vi "Begin.vi"(8 "error in":errorcluster) -> (0 "error out":errorcluster)   [LabVIEW 2018]
doc: "Called before other user functions, this VI can be used to open I/O refnums, load in file data, and do general program initialization. Notice that the <B>error out</B> terminal is simply used for data flow. Wiring it to other structures or subVIs ensures that this VI runs first."
uses:
  <vilib>/Rock Robotics/WPI/DriverStation/WPI_DriverStationRobotMode2.ctl
  <vilib>/Rock Robotics/WPI/Joystick/WPI_JoystickDeviceEnum.ctl
  <vilib>/Rock Robotics/WPI/ThirdParty/Phoenix-LabVIEW/Motor Controller/Controls/CTRE_Phoenix_MotorControl_ControlMode.ctl
  <vilib>/Rock Robotics/WPI/ThirdParty/Phoenix-LabVIEW/Motor Controller/Controls/CTRE_Phoenix_MotorControl_FeedbackDevice.ctl
  <vilib>/Rock Robotics/WPI/ThirdParty/Phoenix-LabVIEW/Motor Controller/Controls/CTRE_Phoenix_MotorControl_NeutralMode.ctl
  <vilib>/Rock Robotics/WPI/SafetyOutput/WPI_SafetyOutputConfigMenu.ctl
  <vilib>/Rock Robotics/SystemInterfaces/DIO/FPGA_DIOChannel.ctl
  Robot Global Data.vi
  <vilib>/Rock Robotics/Network Tables/NT Write String Array.vi
  <vilib>/Rock Robotics/WPI/RobotDrive/WPI_RobotDriveOpen4MotorWithExistingMotors.vi
  <vilib>/Rock Robotics/WPI/RobotDrive/WPI_RobotDriveOpen2MotorWithExistingMotors.vi
  <vilib>/Rock Robotics/WPI/Solenoid/WPI_SolenoidOpenDouble.vi
  <vilib>/Rock Robotics/WPI/Utilities/WPI_GetSetVariantRefNum.vi
  <vilib>/Rock Robotics/WPI/Solenoid/WPI_SolenoidOpenSingle.vi
  <vilib>/Rock Robotics/WPI/Ultrasonic/WPI_SonarSRF04DigitalOpen.vi
  <vilib>/Rock Robotics/WPI/Ultrasonic/WPI_SonarSRF04DigitalRefNum Registry Set.vi
  <vilib>/Rock Robotics/WPI/Switch/WPI_SwitchOpenLimit.vi
panel:
  in  "error in 2":errorcluster
  out "error out 2":errorcluster
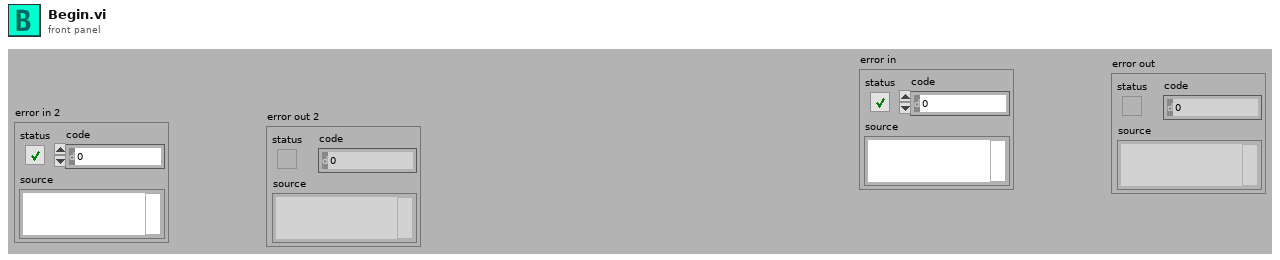
[diagram p1: front panel]
types:
  T1 = typedef "FPGA_DIOChannel.ctl" = enum8{"DIO 0", "DIO 1", "DIO 2", "DIO 3", "DIO 4", "DIO 5", "DIO 6", "DIO 7", "DIO 8", "DIO 9", "DIO MXP 0", "DIO MXP 1", "DIO MXP 2", "DIO MXP 3", "DIO MXP 4", "DIO MXP 5", "DIO MXP 6", "DIO MXP 7", "DIO MXP 8", "DIO MXP 9", "DIO MXP 10", "DIO MXP 11", "DIO MXP 12", "DIO MXP 13", "DIO MXP 14", "DIO MXP 15", "SPI Port CS1", "SPI Port CS2", "SPI Port CS3", "SPI Port MISO", "SPI Port MOSI", "Invalid"}
  T2 = typedef "CTRE_Phoenix_MotorControl_ControlMode.ctl" = u16
  T3 = typedef "WPI_SafetyOutputConfigMenu.ctl" = enum16{"Enable", "Disable"}
  T4 = typedef "WPI_JoystickDeviceEnum.ctl" = enum16{"USB 0", "USB 1", "USB 2", "USB 3", "USB 4", "USB 5"}
  T5 = typedef "CTRE_Phoenix_MotorControl_FeedbackDevice.ctl" = i8
  T6 = typedef "CTRE_Phoenix_MotorControl_NeutralMode.ctl" = enum8{"EEPROMSetting", "Override to Coast", "Override to Brake"}
  T7 = typedef "WPI_DriverStationRobotMode2.ctl" = enum16{"Autonomous Disabled", "Autonomous Enabled", "Teleop Disabled", "Teleop Enabled", "Disconnected", "Finish", "Test Disabled", "Test Enabled", "Emergency Stopped"}
  T8 = typedef "WPI_MotorControlDeviceRef.ctl" = cluster{"DeviceStatus":errorcluster, "Type":T9, "PWM":cluster{"PWM Channel":T10, "DeadBand":T11}, "CAN":cluster{"Device Number":u8, "SetOutput VI Ref":variant, "GetOutput VI Ref":variant, "Enable VI Ref":variant, "Disable VI Ref":variant, "Data":variant}, "Invert":bool, "DIO PWM":cluster{"PWM \"Enable\" Channel":T10, "DIOChannel":T1, "PWM Rate":dbl}}
  T9 = typedef "WPI_MotorControlType.ctl" = enum16{"PWM", "CAN", "DIO PWM"}
  T10 = typedef "FPGA_DIOPWMChannel.ctl" = enum8{"PWM 0", "PWM 1", "PWM 2", "PWM 3", "PWM 4", "PWM 5", "PWM 6", "PWM 7", "PWM 8", "PWM 9", "PWM MXP 0", "PWM MXP 1", "PWM MXP 2", "PWM MXP 3", "PWM MXP 4", "PWM MXP 5", "PWM MXP 6", "PWM MXP 7", "PWM MXP 8", "PWM MXP 9", "Invalid"}
  T11 = typedef "WPI_PWMDeadband.ctl" = cluster{"Name":string, "maxPositivePwm":i32, "minPositivePwm":i32, "centerPwm":i32, "maxNegativePwm":i32, "minNegativePwm":i32, "angularRange":u16}
  T12 = typedef "WPI_JoystickDevRef.ctl" = cluster{"Device":T4}
  T13 = typedef "WPI_CompressorDevRef.ctl" = cluster{"DevStatus":errorcluster, "Pneumatics Control Module":u8}
  T14 = typedef "WPI_SwitchDevRef.ctl" = cluster{"DevStatus":errorcluster, "DIO Channel":T1, "CntIndex":T15, "Normally Closed":bool}
  T15 = typedef "FPGA_CounterCtrSystemIndex.ctl" = enum8{"Ctr 0", "Ctr 1", "Ctr 2", "Ctr 3", "Ctr 4", "Ctr 5", "Ctr 6", "Ctr 7", "Invalid"}
  T16 = typedef "WPI_SolenoidDevRef.ctl" = cluster{"DevStatus":errorcluster, "Pneumatics Control Module":u8, "Forward Solenoid Channel":T17, "Reverse Solenoid Channel":T17}
  T17 = typedef "WPI_SolenoidChannel.ctl" = enum8{"Solenoid 0", "Solenoid 1", "Solenoid 2", "Solenoid 3", "Solenoid 4", "Solenoid 5", "Solenoid 6", "Solenoid 7", "Invalid"}
  T18 = typedef "WPI_RobotDriveDevRef.ctl" = cluster{"DevStatus":errorcluster, "Motors[]":T8[], "Square Inputs":bool, "Max Output":dbl}
  T19 = typedef "WPI_UltrasonicDeviceRef.ctl" = cluster{"DevStatus":errorcluster, "Ping Channel":T1, "Echo Channel":T1, "CntIndex":T15}
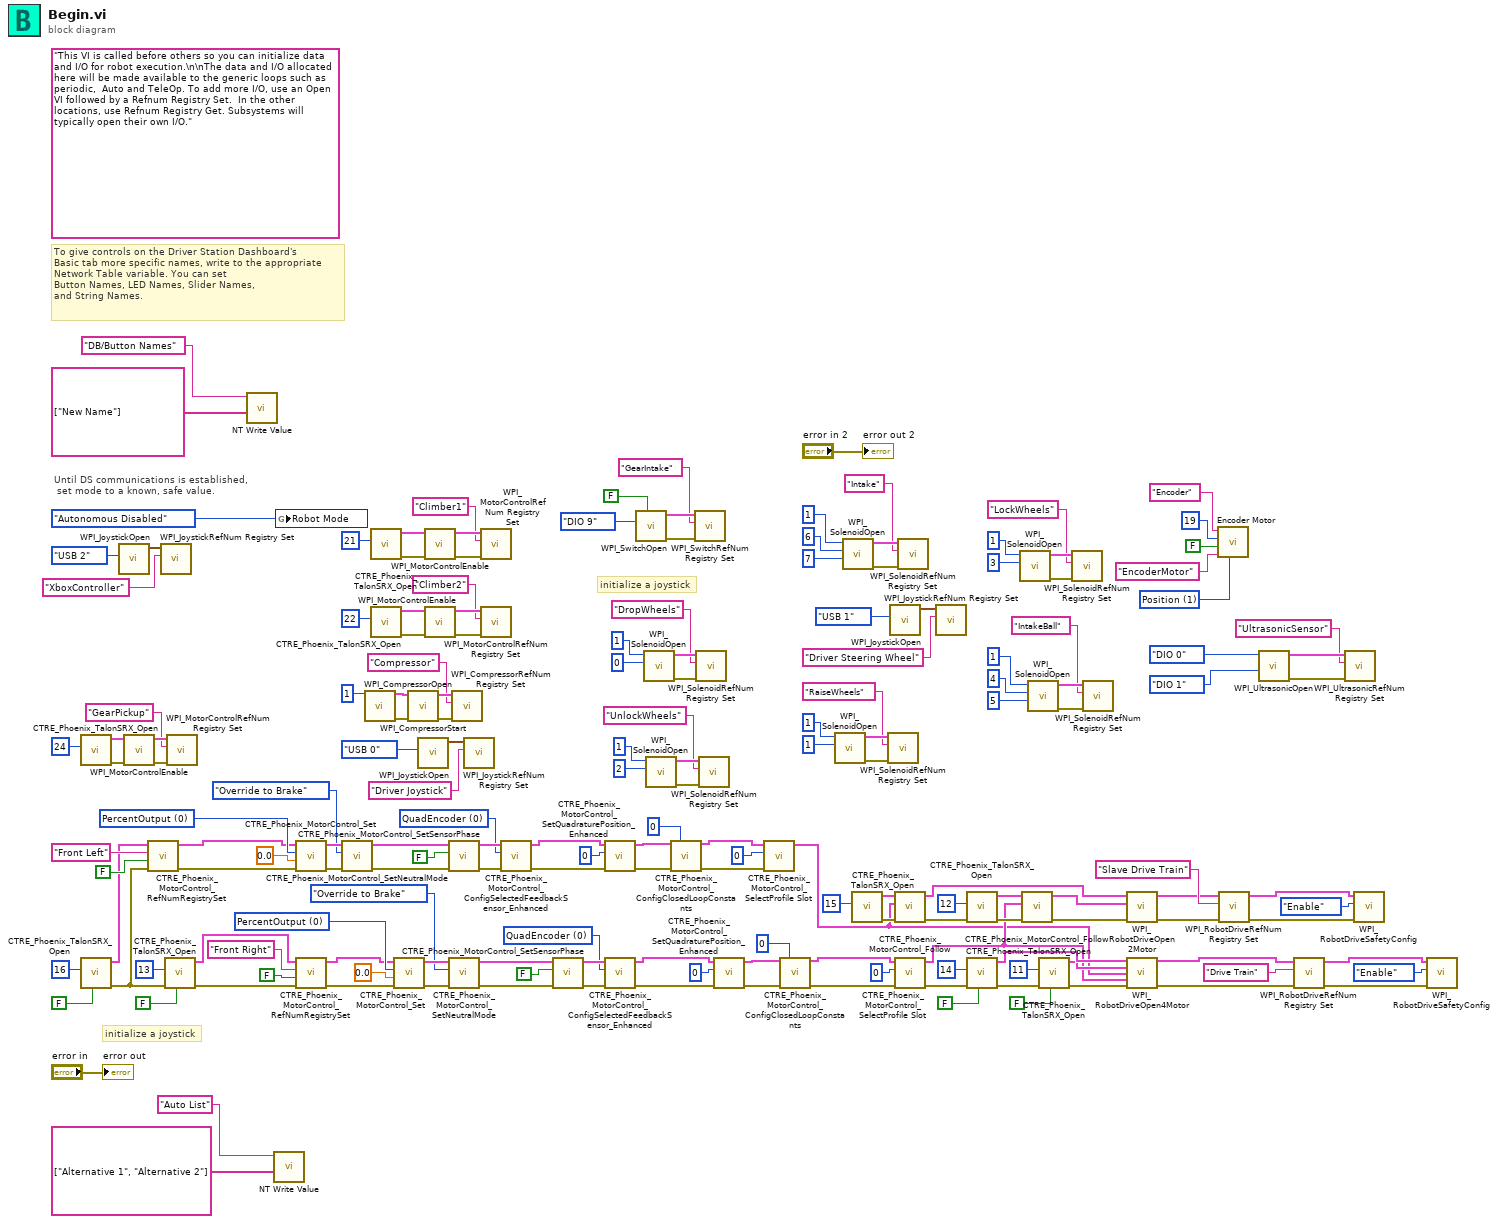
[diagram p0: block diagram]
diagram:
  w1 = T2 1 items=["PercentOutput"=0, "Position"=1, "Velocity"=2, "Current"=3, "Follower"=5, "MotionProfile"=6, "MotionMagic"=7, "MotionMagicArc"=8, "MotionProfileArc"=10, "Disabled"=15] ("Control Mode")
  w111 = T5 0 items=["None"=-1, "QuadEncoder"=0, "Analog"=2, "Tachometer"=4, "Pulse Width Encoded Position"=8, "Sensor Sum (S0 + S1)"=9, "Sensor Difference (D0 - D1)"=10, "Remote Source 0"=11, "Remote Source 1"=12, "Software Emulated"=15] ("Feedback Device")
  w100 = T2 0 items=["PercentOutput"=0, "Position"=1, "Velocity"=2, "Current"=3, "Follower"=5, "MotionProfile"=6, "MotionMagic"=7, "MotionMagicArc"=8, "MotionProfileArc"=10, "Disabled"=15] ("Control Mode")
  w138 = T5 0 items=["None"=-1, "QuadEncoder"=0, "Analog"=2, "Tachometer"=4, "Pulse Width Encoded Position"=8, "Sensor Sum (S0 + S1)"=9, "Sensor Difference (D0 - D1)"=10, "Remote Source 0"=11, "Remote Source 1"=12, "Software Emulated"=15] ("Feedback Device")
  w127 = T2 0 items=["PercentOutput"=0, "Position"=1, "Velocity"=2, "Current"=3, "Follower"=5, "MotionProfile"=6, "MotionMagic"=7, "MotionMagicArc"=8, "MotionProfileArc"=10, "Disabled"=15] ("Control Mode")
  (unwired) "This VI is called before others so you can initialize data and I/O for robot execution.\n\nThe data and I/O allocated here will be made available to the generic loops such as periodic,  Auto and TeleOp. To add more I/O, use an Open VI followed by a Refnum Registry Set.  In the other locations, use Refnum Registry Get. Subsystems will typically open their own I/O."
  # "initialize a joystick"
  # "To give controls on the Driver Station Dashboard's\nBasic tab more specific names, write to the appropriate\nNetwork Table variable. You can set\nButton Names, LED Names, Slider Names,\nand String Names."
  # "initialize a joystick"
  # "Until DS communications is established,\n set mode to a known, safe value."
  n1 = call <vilib>:"CTRE_Phoenix_TalonSRX_Open.vi"("Device Number"=24) -> ("error out"=w70:errorcluster, "CAN Talon SRX Ref"=w69:T8)  [unwired: 9 in]
  n2 = call <vilib>:"CTRE_Phoenix_TalonSRX_Open.vi"("Invert"=FALSE, "Device Number"=u8 16) -> ("error out"=w96:errorcluster, "CAN Talon SRX Ref"=w120:T8)  [unwired: 8 in]
  n3 = call <vilib>:"WPI_JoystickOpen.vi"("JoystickDevice"=WPI_JoystickDeviceEnum."USB 2") -> ("JoystickDevRef"=w91:T12)  [unwired: 10 in]
  n4 = call <vilib>:"WPI_MotorControlEnable.vi"("error in (no error)"=w70, "CAN MotorDevRef"=w69) -> ("error out"=w68:errorcluster, "CAN MotorDevRef"=w67:T8)  [unwired: 8 in]
  n5 = call <vilib>:"CTRE_Phoenix_MotorControl_RefNumRegistrySet.vi"("error in (no error)"=w96, "Test Mode Only"=FALSE, "refnum name"="Front Left", "PhoenixMotorControlDevRef"=w120) -> ("error out"=w98:errorcluster, "PhoenixMotorControlDevRef"=w99:T8)  [unwired: 6 in]
  n6 = call <vilib>:"WPI_JoystickRefNum Registry Set.vi"("refnum name"="XboxController", "JoystickDevRef"=w91) -> ()  [unwired: 8 in, 2 out]
  n7 = call <vilib>:"CTRE_Phoenix_TalonSRX_Open.vi"("Invert"=FALSE, "error in"=w96, "Device Number"=u8 13) -> ("error out"=w147:errorcluster, "CAN Talon SRX Ref"=w148:T8)  [unwired: 7 in]
  n8 = call <vilib>:"WPI_MotorControlRefNum Registry Set.vi"("error in (no error)"=w68, "refnum name"="GearPickup", "MotorControlDevRef"=w67) -> ()  [unwired: 7 in, 2 out]
  n9 = call-poly <vilib>:"NT Write Value.vi"("String Array"=string[] ["New Name"], "Name"="DB/Button Names") -> ()  [unwired: 9 in, 1 out]
  n10 = call-poly <vilib>:"NT Write Value.vi"("String Array"=string[] ["Alternative 1", "Alternative 2"], "Name"="Auto List") -> ()  [unwired: 9 in, 1 out]
  n11 = global write "Robot Global Data.vi" "Robot Mode"(WPI_DriverStationRobotMode2."Autonomous Disabled" ("Robot Mode")) -> ()
  n12 = call <vilib>:"CTRE_Phoenix_MotorControl_Set.vi"("error in (no error)"=w98, "Output"=0.0, "Control Mode"=w100, "PhoenixMotorControlDevRef"=w99) -> ("error out"=w115:errorcluster, "PhoenixMotorControlDevRef"=w119:T8)  [unwired: 6 in]
  n13 = call <vilib>:"CTRE_Phoenix_MotorControl_RefNumRegistrySet.vi"("error in (no error)"=w147, "Test Mode Only"=FALSE, "refnum name"="Front Right", "PhoenixMotorControlDevRef"=w148) -> ("error out"=w125:errorcluster, "PhoenixMotorControlDevRef"=w126:T8)  [unwired: 6 in]
  n14 = call <vilib>:"CTRE_Phoenix_MotorControl_SetNeutralMode.vi"("error in (no error)"=w115, "Motor Control Neutral Mode"=CTRE_Phoenix_MotorControl_NeutralMode."Override to Brake", "PhoenixMotorControlDevRef"=w119) -> ("error out"=w117:errorcluster, "PhoenixMotorControlDevRef"=w116:T8)  [unwired: 7 in]
  n15 = call <vilib>:"WPI_CompressorOpen.vi"("Pneumatics Control Module (0)"=1) -> ("CompressorDevRef"=w58:T13, "error out"=w59:errorcluster)  [unwired: 13 in]
  n16 = call <vilib>:"CTRE_Phoenix_TalonSRX_Open.vi"("Device Number"=21) -> ("error out"=w32:errorcluster, "CAN Talon SRX Ref"=w31:T8)  [unwired: 9 in]
  n17 = call <vilib>:"CTRE_Phoenix_TalonSRX_Open.vi"("Device Number"=22) -> ("error out"=w26:errorcluster, "CAN Talon SRX Ref"=w25:T8)  [unwired: 9 in]
  n18 = call <vilib>:"CTRE_Phoenix_MotorControl_Set.vi"("error in (no error)"=w125, "Output"=0.0, "Control Mode"=w127, "PhoenixMotorControlDevRef"=w126) -> ("error out"=w142:errorcluster, "PhoenixMotorControlDevRef"=w146:T8)  [unwired: 6 in]
  n19 = call <vilib>:"WPI_CompressorStart.vi"("error in (no error)"=w59, "CompressorDevRef"=w58) -> ("error out"=w57:errorcluster, "CompressorDevRef"=w56:T13)  [unwired: 8 in]
  n20 = call <vilib>:"WPI_JoystickOpen.vi"("JoystickDevice"=WPI_JoystickDeviceEnum."USB 0") -> ("JoystickDevRef"=w169:T12)  [unwired: 10 in]
  n21 = call <vilib>:"WPI_MotorControlEnable.vi"("error in (no error)"=w32, "CAN MotorDevRef"=w31) -> ("error out"=w30:errorcluster, "CAN MotorDevRef"=w29:T8)  [unwired: 8 in]
  n22 = call <vilib>:"WPI_MotorControlEnable.vi"("error in (no error)"=w26, "CAN MotorDevRef"=w25) -> ("error out"=w24:errorcluster, "CAN MotorDevRef"=w23:T8)  [unwired: 8 in]
  n23 = call <vilib>:"CTRE_Phoenix_MotorControl_SetSensorPhase.vi"("error in (no error)"=w117, "PhaseSensor"=FALSE, "PhoenixMotorControlDevRef"=w116) -> ("error out"=w113:errorcluster, "PhoenixMotorControlDevRef"=w112:T8)  [unwired: 7 in]
  n24 = call <vilib>:"CTRE_Phoenix_MotorControl_SetNeutralMode.vi"("error in (no error)"=w142, "Motor Control Neutral Mode"=CTRE_Phoenix_MotorControl_NeutralMode."Override to Brake", "PhoenixMotorControlDevRef"=w146) -> ("error out"=w144:errorcluster, "PhoenixMotorControlDevRef"=w143:T8)  [unwired: 7 in]
  n25 = call <vilib>:"WPI_CompressorRefNum Registry Set.vi"("error in (no error)"=w57, "refnum name"="Compressor", "CompressorDevRef"=w56) -> ()  [unwired: 7 in, 2 out]
  n26 = call <vilib>:"WPI_JoystickRefNum Registry Set.vi"("refnum name"="Driver Joystick", "JoystickDevRef"=w169) -> ()  [unwired: 8 in, 2 out]
  n27 = call <vilib>:"WPI_MotorControlRefNum Registry Set.vi"("error in (no error)"=w30, "refnum name"="Climber1", "MotorControlDevRef"=w29) -> ()  [unwired: 7 in, 2 out]
  n28 = call <vilib>:"WPI_MotorControlRefNum Registry Set.vi"("error in (no error)"=w24, "refnum name"="Climber2", "MotorControlDevRef"=w23) -> ()  [unwired: 7 in, 2 out]
  n29 = call <vilib>:"CTRE_Phoenix_MotorControl_ConfigSelectedFeedbackSensor_Enhanced.vi"("error in (no error)"=w113, "Feedback Device"=w111, "PhoenixMotorControlDevRef"=w112) -> ("error out"=w109:errorcluster, "PhoenixMotorControlDevRef"=w110:T8)  [unwired: 7 in]
  n30 = call <vilib>:"CTRE_Phoenix_MotorControl_SetSensorPhase.vi"("error in (no error)"=w144, "PhaseSensor"=FALSE, "PhoenixMotorControlDevRef"=w143) -> ("error out"=w140:errorcluster, "PhoenixMotorControlDevRef"=w139:T8)  [unwired: 7 in]
  n31 = call <vilib>:"CTRE_Phoenix_MotorControl_SetQuadraturePosition_Enhanced.vi"("error in (no error)"=w109, "New Position"=0, "PhoenixMotorControlDevRef"=w110) -> ("error out"=w106:errorcluster, "PhoenixMotorControlDevRef"=w107:T8)  [unwired: 7 in]
  n32 = call <vilib>:"CTRE_Phoenix_MotorControl_ConfigSelectedFeedbackSensor_Enhanced.vi"("error in (no error)"=w140, "Feedback Device"=w138, "PhoenixMotorControlDevRef"=w139) -> ("error out"=w136:errorcluster, "PhoenixMotorControlDevRef"=w137:T8)  [unwired: 7 in]
  n33 = call-poly <vilib>:"WPI_SwitchOpen.vi"("Normally Closed"=FALSE, "DIO Channel"=FPGA_DIOChannel."DIO 9") -> ("error out"=w10:errorcluster, "SwitchDevRef"=w9:T14)  [unwired: 8 in]
  n34 = call-poly <vilib>:"WPI_SolenoidOpen.vi"("Solenoid Channel"=u8 0 ("Pneumatics Control Module (0)"), "Pneumatics Control Module (0)"=u8 1) -> ("error out"=w46:errorcluster, "SolenoidDevRef"=w47:T16)  [unwired: 8 in]
  n35 = call-poly <vilib>:"WPI_SolenoidOpen.vi"("Solenoid Channel"=u8 2 ("Pneumatics Control Module (0)"), "Pneumatics Control Module (0)"=u8 1) -> ("error out"=w41:errorcluster, "SolenoidDevRef"=w42:T16)  [unwired: 8 in]
  n36 = call <vilib>:"CTRE_Phoenix_MotorControl_ConfigClosedLoopConstants.vi"("PhoenixMotorControlDevRef"=w107, "slotIdx"=0, "error in (no error)"=w106) -> ("PhoenixMotorControlDevRef"=w103:T8, "error out"=w104:errorcluster)  [unwired: 11 in]
  n37 = call <vilib>:"WPI_SwitchRefNum Registry Set.vi"("error in (no error)"=w10, "refnum name"="GearIntake", "SwitchDevRef"=w9) -> ()  [unwired: 7 in, 2 out]
  n38 = call <vilib>:"WPI_SolenoidRefNum Registry Set.vi"("error in (no error)"=w46, "refnum name"="DropWheels", "SolenoidDevRef"=w47) -> ()  [unwired: 7 in, 2 out]
  n39 = call <vilib>:"WPI_SolenoidRefNum Registry Set.vi"("error in (no error)"=w41, "refnum name"="UnlockWheels", "SolenoidDevRef"=w42) -> ()  [unwired: 7 in, 2 out]
  n40 = call <vilib>:"CTRE_Phoenix_MotorControl_SetQuadraturePosition_Enhanced.vi"("error in (no error)"=w136, "New Position"=0, "PhoenixMotorControlDevRef"=w137) -> ("error out"=w133:errorcluster, "PhoenixMotorControlDevRef"=w134:T8)  [unwired: 7 in]
  n41 = call <vilib>:"CTRE_Phoenix_MotorControl_SelectProfile Slot.vi"("error in (no error)"=w104, "slotIdx"=0, "PhoenixMotorControlDevRef"=w103) -> ("PhoenixMotorControlDevRef"=w72:T8)  [unwired: 7 in, 1 out]
  n42 = call <vilib>:"CTRE_Phoenix_MotorControl_ConfigClosedLoopConstants.vi"("PhoenixMotorControlDevRef"=w134, "slotIdx"=0, "error in (no error)"=w133) -> ("PhoenixMotorControlDevRef"=w130:T8, "error out"=w131:errorcluster)  [unwired: 11 in]
  n43 = call-poly <vilib>:"WPI_SolenoidOpen.vi"("Solenoid Channel"=u8 1 ("Pneumatics Control Module (0)"), "Pneumatics Control Module (0)"=u8 1) -> ("error out"=w50:errorcluster, "SolenoidDevRef"=w51:T16)  [unwired: 8 in]
  n44 = call-poly <vilib>:"WPI_SolenoidOpen.vi"("Reverse Solenoid Channel"=7, "Forward Solenoid Channel"=6, "Pneumatics Control Module (0)"=1) -> ("error out"=w62:errorcluster, "SolenoidDevRef"=w63:T16)  [unwired: 7 in]
  n45 = call <vilib>:"CTRE_Phoenix_TalonSRX_Open.vi"("Device Number"=15) -> ("error out"=w88:errorcluster, "CAN Talon SRX Ref"=w89:T8)  [unwired: 9 in]
  n46 = call <vilib>:"WPI_SolenoidRefNum Registry Set.vi"("error in (no error)"=w50, "refnum name"="RaiseWheels", "SolenoidDevRef"=w51) -> ()  [unwired: 7 in, 2 out]
  n47 = call <vilib>:"WPI_JoystickOpen.vi"("JoystickDevice"=WPI_JoystickDeviceEnum."USB 1") -> ("JoystickDevRef"=w153:T12)  [unwired: 10 in]
  n48 = call <vilib>:"CTRE_Phoenix_MotorControl_Follow.vi"("error in (no error)"=w88, "Master Controller to Follow"=w72, "PhoenixMotorControlDevRef"=w89) -> ("error out"=w77:errorcluster, "PhoenixMotorControlDevRef"=w81:T8)  [unwired: 7 in]
  n49 = call <vilib>:"CTRE_Phoenix_MotorControl_SelectProfile Slot.vi"("error in (no error)"=w131, "slotIdx"=0, "PhoenixMotorControlDevRef"=w130) -> ("error out"=w95:errorcluster, "PhoenixMotorControlDevRef"=w75:T8)  [unwired: 7 in]
  n50 = call <vilib>:"WPI_SolenoidRefNum Registry Set.vi"("error in (no error)"=w62, "refnum name"="Intake", "SolenoidDevRef"=w63) -> ()  [unwired: 7 in, 2 out]
  n51 = call <vilib>:"WPI_JoystickRefNum Registry Set.vi"("refnum name"="Driver Steering Wheel", "JoystickDevRef"=w153) -> ()  [unwired: 8 in, 2 out]
  n52 = call <vilib>:"CTRE_Phoenix_TalonSRX_Open.vi"("error in"=w77, "Device Number"=12) -> ("error out"=w79:errorcluster, "CAN Talon SRX Ref"=w80:T8)  [unwired: 8 in]
  n53 = call <vilib>:"CTRE_Phoenix_TalonSRX_Open.vi"("Invert"=FALSE, "error in"=w95, "Device Number"=14) -> ("error out"=w94:errorcluster, "CAN Talon SRX Ref"=w166:T8)  [unwired: 7 in]
  n54 = call-poly <vilib>:"WPI_SolenoidOpen.vi"("Solenoid Channel"=u8 3 ("Pneumatics Control Module (0)"), "Pneumatics Control Module (0)"=u8 1) -> ("error out"=w36:errorcluster, "SolenoidDevRef"=w37:T16)  [unwired: 8 in]
  n55 = call <vilib>:"CTRE_Phoenix_MotorControl_Follow.vi"("error in (no error)"=w79, "Master Controller to Follow"=w75, "PhoenixMotorControlDevRef"=w80) -> ("error out"=w76:errorcluster, "PhoenixMotorControlDevRef"=w78:T8)  [unwired: 7 in]
  n56 = call-poly <vilib>:"WPI_SolenoidOpen.vi"("Reverse Solenoid Channel"=5, "Forward Solenoid Channel"=4, "Pneumatics Control Module (0)"=1) -> ("error out"=w13:errorcluster, "SolenoidDevRef"=w14:T16)  [unwired: 7 in]
  n57 = call <vilib>:"CTRE_Phoenix_TalonSRX_Open.vi"("Invert"=FALSE, "error in"=w94, "Device Number"=11) -> ("error out"=w93:errorcluster, "CAN Talon SRX Ref"=w165:T8)  [unwired: 7 in]
  n58 = call <vilib>:"WPI_SolenoidRefNum Registry Set.vi"("error in (no error)"=w36, "refnum name"="LockWheels", "SolenoidDevRef"=w37) -> ()  [unwired: 7 in, 2 out]
  n59 = call <vilib>:"WPI_SolenoidRefNum Registry Set.vi"("error in (no error)"=w13, "refnum name"="IntakeBall", "SolenoidDevRef"=w14) -> ()  [unwired: 7 in, 2 out]
  n60 = call-poly <vilib>:"WPI_RobotDriveOpen2Motor.vi"("error in (no error)"=w76, "Right Motor Dev Ref"=w78, "Left Motor Dev Ref"=w81) -> ("error out"=w82:errorcluster, "RobotDriveDevRef"=w83:T18)  [unwired: 7 in]
  n61 = call-poly <vilib>:"WPI_RobotDriveOpen4Motor.vi"("Rear Left Motor Dev Ref"=w166, "Rear Right Motor Dev Ref"=w165, "Front Left Motor Dev Ref"=w72, "Front Right Motor Dev Ref"=w75, "error in (no error)"=w93) -> ("RobotDriveDevRef"=w164:T18, "error out"=w163:errorcluster)  [unwired: 9 in]
  n62 = call "Encoder Motor.vi"("Count Type"=w1, "Motor Refnum"="EncoderMotor", "Inversion"=FALSE ("Invert"), "CAN ID"=u8 19 ("Device Number"), "Encoder Refnum"="Encoder") -> ()  [unwired: 7 in]
  n63 = call <vilib>:"WPI_RobotDriveRefNum Registry Set.vi"("error in (no error)"=w82, "refnum name"="Slave Drive Train", "RobotDriveDevRef"=w83) -> ("error out"=w85:errorcluster, "RobotDriveDevRef"=w86:T18)  [unwired: 7 in]
  n64 = call-poly <vilib>:"WPI_UltrasonicOpen.vi"("Echo DIO Channel"=FPGA_DIOChannel."DIO 1", "Ping DIO Channel"=FPGA_DIOChannel."DIO 0") -> ("error out"=w20:errorcluster, "SonarSRF04DevRef"=w21:T19)  [unwired: 8 in]
  n65 = call <vilib>:"WPI_RobotDriveRefNum Registry Set.vi"("error in (no error)"=w163, "refnum name"="Drive Train", "RobotDriveDevRef"=w164) -> ("error out"=w156:errorcluster, "RobotDriveDevRef"=w157:T18)  [unwired: 7 in]
  n66 = call-poly <vilib>:"WPI_UltrasonicRefNum Registry Set.vi"("error in (no error)"=w20, "refnum name"="UltrasonicSensor", "SonarSRF04DevRef"=w21) -> ()  [unwired: 7 in, 2 out]
  n67 = call <vilib>:"WPI_RobotDriveSafetyConfig.vi"("error in (no error)"=w85, "mode"=WPI_SafetyOutputConfigMenu."Enable", "RobotDriveDevRef"=w86) -> ()  [unwired: 7 in, 2 out]
  n68 = call <vilib>:"WPI_RobotDriveSafetyConfig.vi"("error in (no error)"=w156, "mode"=WPI_SafetyOutputConfigMenu."Enable", "RobotDriveDevRef"=w157) -> ()  [unwired: 7 in, 2 out]
  "error out" <- "error in"
  "error out 2" <- "error in 2"
